vi "G#Interface_GetInstance.vi"(0 "reference in":refnum<class "G#Interface.lvclass">, 5 "error in (no error)":errorcluster) -> (14 "reference out":refnum<class "G#Interface.lvclass">, 15 "not a refnum?":bool, 16 "G#Object":refnum<class "G#Object.lvclass">, 19 "error out":errorcluster)   [LabVIEW 2020, in "G#Interface.lvclass"]
doc: "Returns the instance to the G#Object that is wrapped behind the interface."
uses:
  G#Interface.lvclass
  G#Object/G#Object.lvclass
  G#Interface.lvclass/G#Interface.ctl
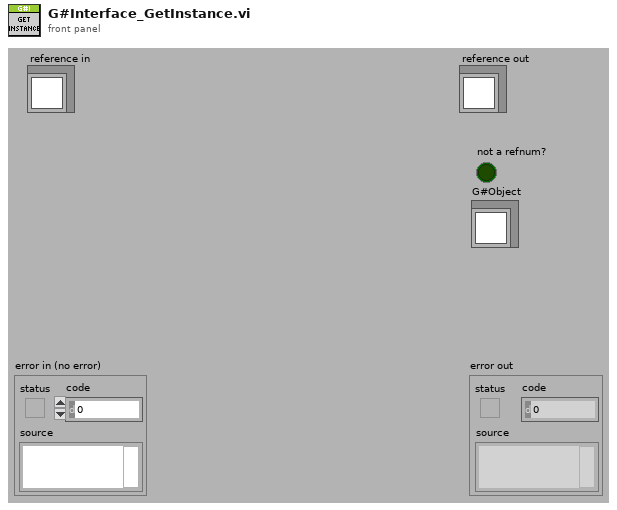
[diagram p1: front panel]
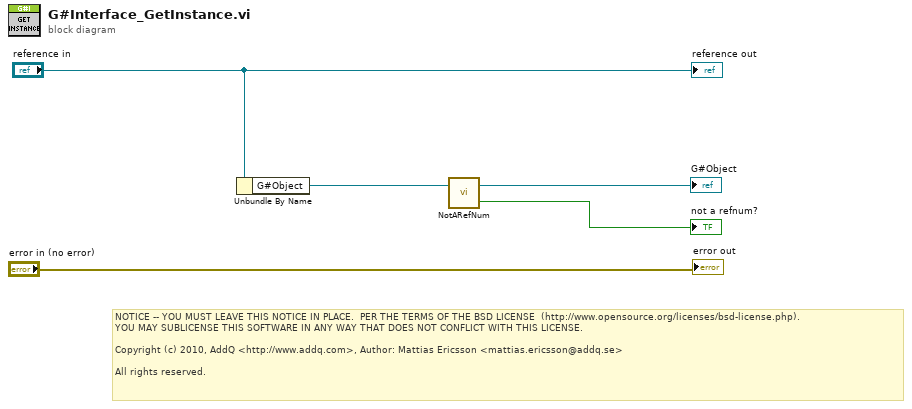
[diagram p0: block diagram]
diagram:
  # "NOTICE -- YOU MUST LEAVE THIS NOTICE IN PLACE.  PER THE TERMS OF THE BSD LICENSE  (http://www.opensource.org/licenses/bsd-license.php).\nYOU MAY SUBLICENSE THIS SOFTWARE IN ANY WAY THAT DOES NOT CONFLICT WITH THIS LICENSE.\n\nCopyright (c) 2010, AddQ <http://www.addq.com>, Author: Mattias Ericsson <mattias.ericsson@addq.se>\n\nAll rights reserved."
  n1 = Unbundle By Name("reference in") -> ("G#Object"=w3:refnum<class "G#Object.lvclass">)
  n2 = call-dynamic "NotARefNum.vi"("reference in"=w3) -> ("not a refnum?"=→"not a refnum?":bool, "reference out"=→"G#Object":refnum<class "G#Object.lvclass">)  [unwired: 1 in]
  "error out" <- "error in (no error)"
  "reference out" <- "reference in"
